vi "Main.vi"(11 "Module Admin":refnum<class "Delacor_lib_QMH_Module Admin.lvclass">) -> ()   [LabVIEW 2019, in "ManejoArchivos.lvlib"]
doc: "This template is based off of the Queued Message Handler design pattern and the Queued Message Handler project template that ships with LabVIEW.\n\nThe main difference is that the queue is private to this module and communication between modules is performed via Broadcast and Request events.\n\nRequest events are wrapped in public API methods and are handled in the Event Handling Loop (EHL) of this VI. Any module can register for Broadcast events sent by this module. The EHL generates messages based on user interface actions.\n\nThe Message Handling Loop (MHL) processes messages generated by the EHL, or by other messages. The messages are string values, so new messages can be added easily to the Message Cases case structure in the MHL. Each message cluster can also provide an optional value for Message Data, which is a variant that can be converted to whatever message-specific data is required.\n_____\nBased on DQMH Dev Tools: Project Template 7.1.0.1490."
uses:
  ManejoArchivos.lvlib
  <vilib>/Delacor/Delacor QMH/Libraries/Module Admin_class/Delacor_lib_QMH_Module Admin.lvclass
  Module Data--cluster.ctl
  Class Definitions/File/File.lvclass
  <vilib>/Delacor/Delacor QMH/Libraries/Message Queue_class/Delacor_lib_QMH_Message Queue.lvclass/Delacor_lib_QMH_Message Queue.ctl
  Stop Argument--cluster.ctl
  <vilib>/Delacor/Delacor QMH/Libraries/Module Admin_class/Delacor_lib_QMH_Module Admin.lvclass/Delacor_lib_QMH_Module Admin.ctl
  Set Column Headers Argument--cluster.ctl
  View File Argument--cluster.ctl
  Set File Path Argument--cluster.ctl
  Set File Settings Argument--cluster.ctl
  Log Data Argument--cluster.ctl
  Log Data (Reply Payload)--cluster.ctl
  Set File Format Argument--cluster.ctl
  File Formats--enum.ctl
  Close File Argument--cluster.ctl
  Get Number of Columns Argument--cluster.ctl
  Get Number of Columns (Reply Payload)--cluster.ctl
  <vilib>/Utility/miscctls.llb/LVPointTypeDef.ctl
  Class Definitions/File/File.lvclass/File.ctl
  <vilib>/Delacor/Delacor QMH/Libraries/Message Queue_class/Delacor_lib_QMH_Enqueue Message (Single).vi
  <vilib>/Delacor/Delacor QMH/Libraries/Module Admin_class/Delacor_lib_QMH_Get External Launch.vi
  Class Definitions/File/Write Column Headers.vi
  Class Definitions/File/Write File Path.vi
  Class Definitions/File/Write Save Timestamp.vi
  Class Definitions/File/Write Delimiter.vi
  Class Definitions/File/Read Column Headers.vi
  <vilib>/Delacor/Delacor QMH/Libraries/Message Queue_class/Delacor_lib_QMH_Message Queue.lvclass
panel:
  out "error out":errorcluster
  out "Status":string
  in  "Simulate MHL Error":bool
  in  "Simulate EHL Error":bool
  # "Other processes communicate with this Module via its Public API (wrappers for its Request Events).\n\nThis Module communicates with other processes via its Broadcast Events.\nAny process that wants to receive these messages can register for this module's Broadcast events."
  # "This template is for the DQMH framework. See the block diagram for more information on how to use this template."
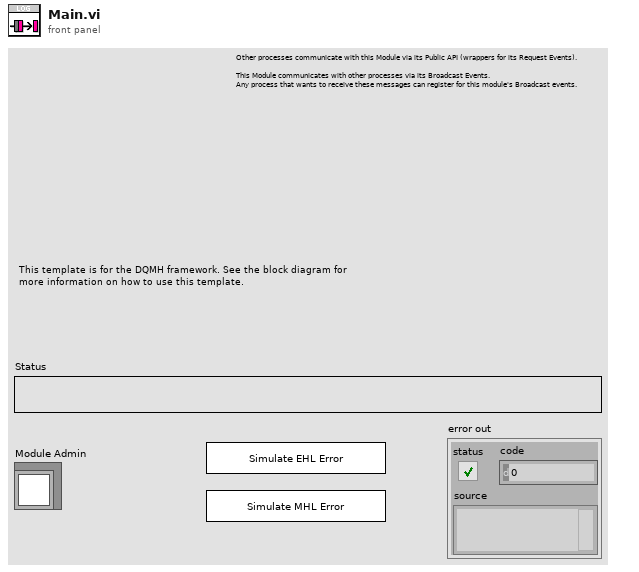
[diagram p1: front panel]
types:
  T1 = typedef "ManejoArchivos.lvlib/Request Events--cluster.ctl" = cluster{"Stop Module":refnum<user-event>, "Show Panel":refnum<user-event>, "Hide Panel":refnum<user-event>, "Get Module Execution Status":refnum<user-event>, "Show Diagram":refnum<user-event>, "Set Column Headers":refnum<user-event>, "View File":refnum<user-event>, "Set File Path":refnum<user-event>, "Set File Settings":refnum<user-event>, "Log Data":refnum<user-event>, "Set File Format":refnum<user-event>, "Close File":refnum<user-event>, "Get Number of Columns":refnum<user-event>}
  T2 = typedef "ManejoArchivos.lvlib/Module Data--cluster.ctl" = cluster{"Status":string, "File Obj":refnum<class "File.lvclass">, "View File":bool}
  T3 = enum32{"invalid lock state", "Not Locked", "Locked (No Password)", "Password-protected"}
  T4 = typedef "ManejoArchivos.lvlib/Stop Argument--cluster.ctl" = cluster{"Origin":string, "Exit via Stop Module Req?":bool, "Wait for Module to stop?":bool}
  T5 = typedef "ManejoArchivos.lvlib/Set Column Headers Argument--cluster.ctl" = cluster{"Headers":string[]}
  T6 = typedef "ManejoArchivos.lvlib/View File Argument--cluster.ctl" = cluster{"Boolean":bool}
  T7 = typedef "ManejoArchivos.lvlib/Set File Path Argument--cluster.ctl" = cluster{"Path":path}
  T8 = typedef "ManejoArchivos.lvlib/Set File Settings Argument--cluster.ctl" = cluster{"Save Time Stamp":bool, "Delimiter":enum16{"Tab", "Coma"}}
  T9 = typedef "ManejoArchivos.lvlib/Log Data Argument--cluster.ctl" = cluster{"Data":dbl[], "Wait Notifier":refnum<notifier>, "wait for reply":bool}
  T10 = typedef "ManejoArchivos.lvlib/Set File Format Argument--cluster.ctl" = cluster{"Format":T11}
  T11 = typedef "ManejoArchivos.lvlib/File Formats--enum.ctl" = enum16{"TDMS", "CSV"}
  T12 = typedef "ManejoArchivos.lvlib/Close File Argument--cluster.ctl" = cluster{"Boolean":bool}
  T13 = typedef "ManejoArchivos.lvlib/Get Number of Columns Argument--cluster.ctl" = cluster{"Wait Notifier":refnum<notifier>, "wait for reply":bool}
  T14 = typedef "LVPointTypeDef.ctl" = cluster{"Horizontal":i16, "Vertical":i16}
  T15 = enum32{"Invalid", "Standard", "Closed", "Hidden", "Minimized", "Maximized"}
  T16 = typedef "ManejoArchivos.lvlib/Log Data (Reply Payload)--cluster.ctl" = cluster{"error":errorcluster}
  T17 = typedef "ManejoArchivos.lvlib/Get Number of Columns (Reply Payload)--cluster.ctl" = cluster{"error":errorcluster, "Number Of Columns":i32}
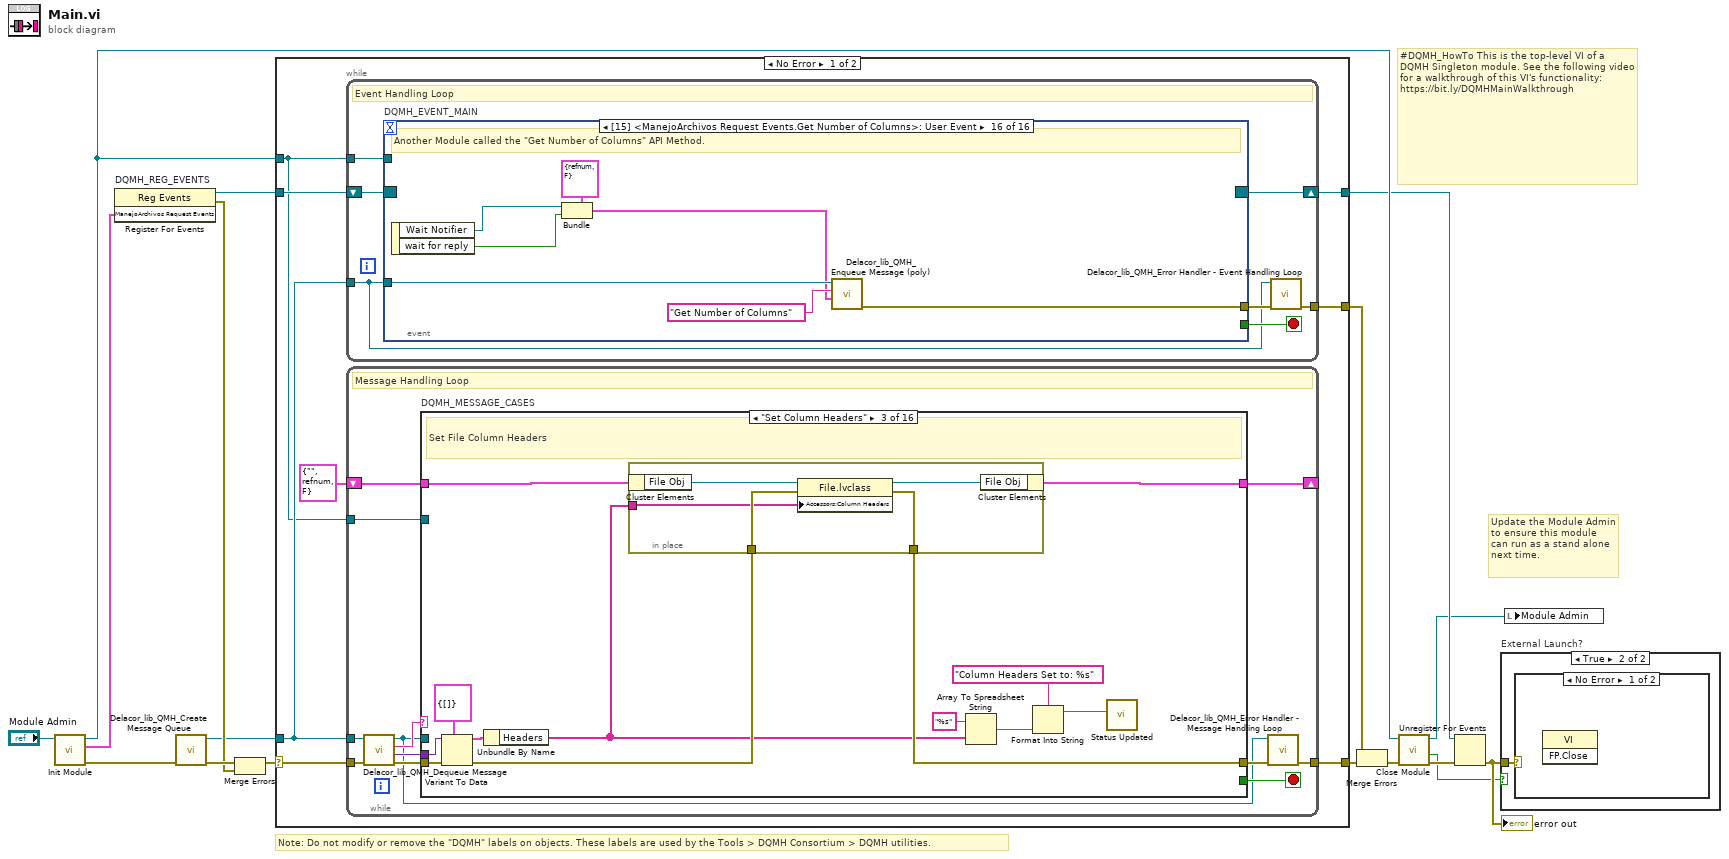
[diagram p0: block diagram]
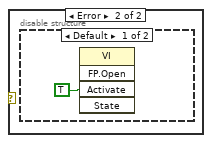
[diagram p3: hidden frame]
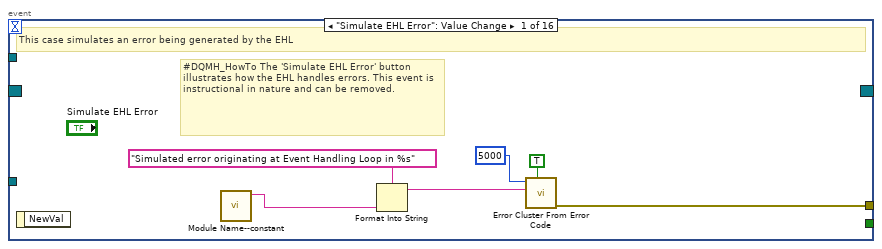
[diagram p5: hidden frame]
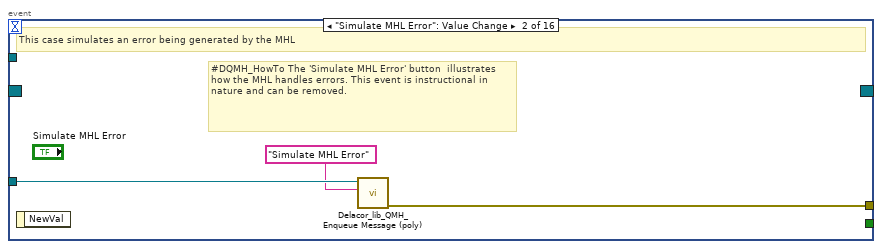
[diagram p6: hidden frame]
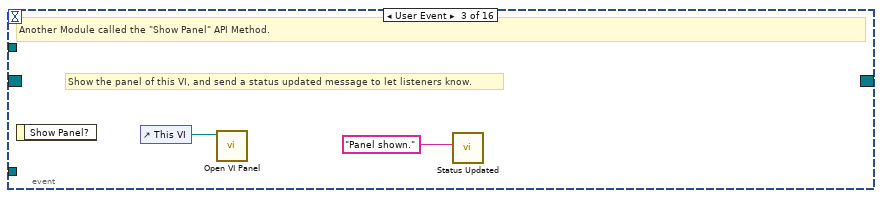
[diagram p7: hidden frame]
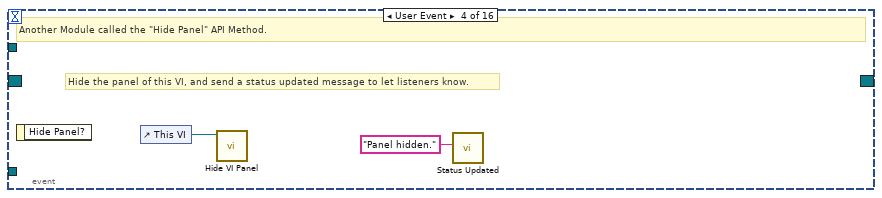
[diagram p8: hidden frame]
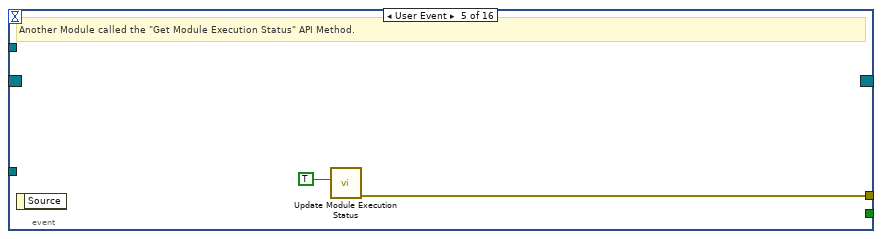
[diagram p9: hidden frame]
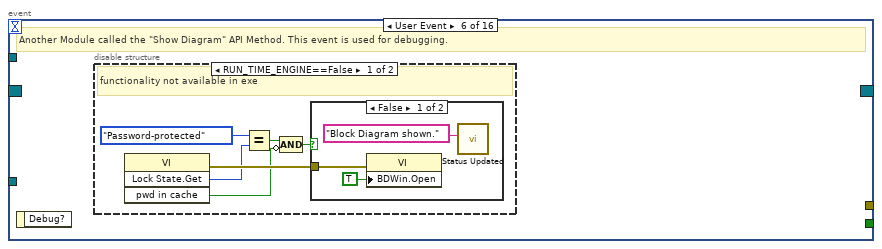
[diagram p10: hidden frame]
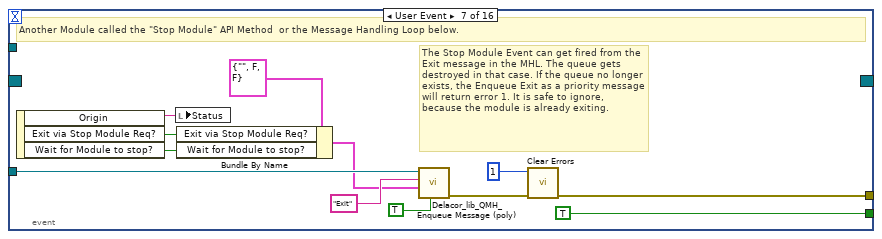
[diagram p13: hidden frame]
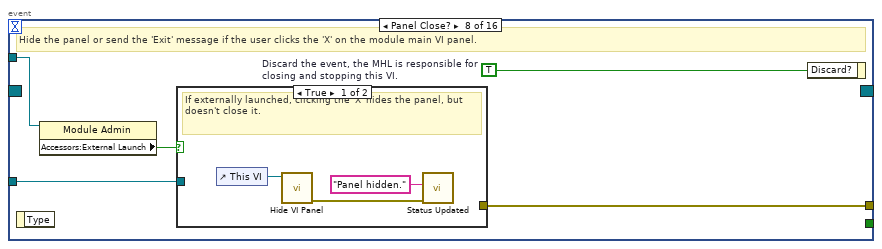
[diagram p14: hidden frame]
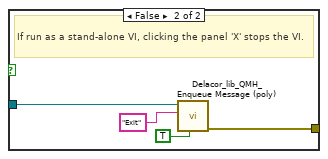
[diagram p15: hidden frame]
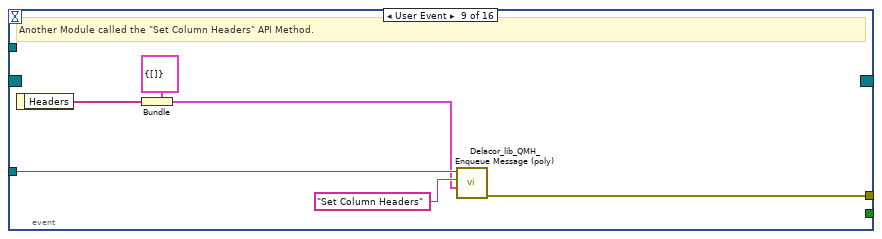
[diagram p16: hidden frame]
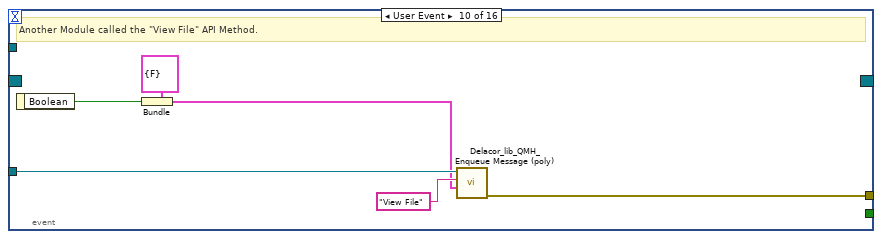
[diagram p17: hidden frame]
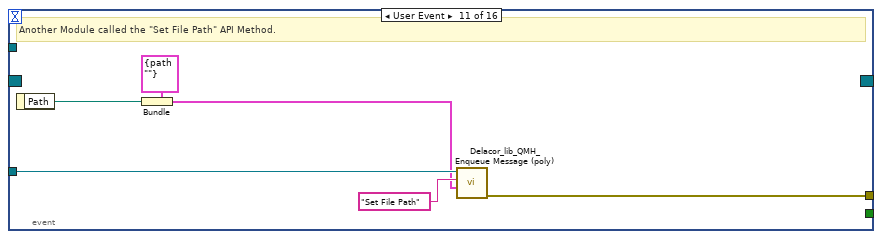
[diagram p18: hidden frame]
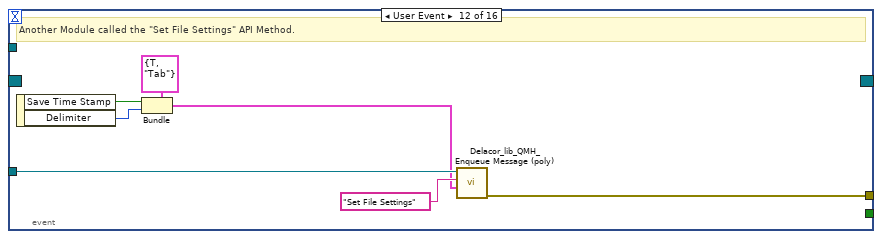
[diagram p19: hidden frame]
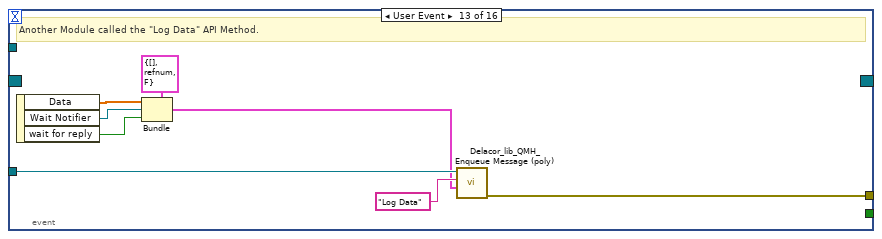
[diagram p20: hidden frame]
diagram:
  # "#DQMH_HowTo This is the top-level VI of a DQMH Singleton module. See the following video for a walkthrough of this VI's functionality: https://bit.ly/DQMHMainWalkthrough"
  # "Note: Do not modify or remove the \"DQMH\" labels on objects. These labels are used by the Tools > DQMH Consortium > DQMH utilities."
  # "Update the Module Admin to ensure this module can run as a stand alone next time."
  n1 = call "Init Module.vi"("Singleton Module Admin in"="Module Admin") -> ("error out"=w16:errorcluster, "ManejoArchivos Request Events"=w5:T1, "Singleton Module Admin out"=w8:refnum<class "Delacor_lib_QMH_Module Admin.lvclass">)  [unwired: 8 in]
  n2 = register-events "DQMH_REG_EVENTS"(w5) -> (reference out=w6:refnum<event-registration>, error out=w9:errorcluster)  [unwired: 2 in]
  n3 = call <vilib>:"Delacor_lib_QMH_Create Message Queue.vi"("error in"=w16) -> ("error out"=w11:errorcluster, "Message Queue"=w4:refnum<class "Delacor_lib_QMH_Message Queue.lvclass">)  [unwired: 9 in]
  n4 = Merge Errors(w11, w9) -> (w10:errorcluster)
  n5 = case shown="No Error" w10 {
    selector: w10 -> [w23 w357]
    tunnel: [w25 w356] -> w17
    tunnel: [w22 w355] -> w7
    tunnel: w6 -> [w20 w355]
    tunnel: w4 -> [w19 w350]
    tunnel: [w24 _] -> w14
    tunnel: w8 -> [w18 w351]
    frame No Error {
      n6 = while {
        tunnel: w19 -> [w26]
        shift-right: [w29] -> w22
        shift-left: w20 -> [w30]
        tunnel: [w31] -> w24
        tunnel: w18 -> [w27]
        stop <- w28 stop-if-true
        # "Event Handling Loop"
        n7 = event "DQMH_EVENT_MAIN" shown="[15] <ManejoArchivos Request Events.Get Number of Columns>: User Event" {
          selector: w30 -> [_ _ _ _ _ _ _ _ _ _ _ _ _ _ _ _]
          dyn-events: [_ _ _ _ _ _ _ _ _ _ _ _ _ _ _ _] -> w29
          timeout: _ -> [_ _ _ _ _ _ _ _ _ _ _ _ _ _ _ _]
          tunnel: [_ _ _ _ _ _ TRUE ("Discard?") _ _ _ _ _ _ _ _ _] -> w28
          tunnel: w26 -> [_ w40 _ _ _ _ w64 w71 w86 w92 w98 w105 w113 w119 w125 w132]
          tunnel: [w38 w41 _ _ w47 _ w67 w73 w81 w87 w93 w99 w108 w114 w120 w128] -> w32
          tunnel: w27 -> [_ _ _ _ _ _ _ w70 _ _ _ _ _ _ _ _]
          event "Simulate EHL Error": Value Change {
            # "#DQMH_HowTo The 'Simulate EHL Error' button  illustrates how the EHL handles errors. This event is instructional in nature and can be removed."
            # "This case simulates an error being generated by the EHL"
            n8 = event-data() -> ()  [unwired: 1 in, 1 out]
            n9 = call "Module Name--constant.vi"() -> ("Module Name"=w35:string)  [unwired: 11 in]
            n10 = Format Into String(format string="Simulated error originating at Event Handling Loop in %s", w35) -> (resulting string=w36:string)  [unwired: 2 in, 1 out]
            n11 = call <vilib>:"Error Cluster From Error Code.vi"("show call chain? (False)"=TRUE, "error message (\"\")"=w36, "error code (0)"=5000) -> ("error out"=w38:errorcluster)  [unwired: 6 in]
          }
          event "Simulate MHL Error": Value Change {
            # "#DQMH_HowTo The 'Simulate MHL Error' button  illustrates how the MHL handles errors. This event is instructional in nature and can be removed."
            # "This case simulates an error being generated by the MHL"
            n12 = event-data() -> ()  [unwired: 1 in, 1 out]
            n13 = call-poly <vilib>:"Delacor_lib_QMH_Enqueue Message (poly).vi"("Message"="Simulate MHL Error", "Message Queue in"=w40) -> ("error out"=w41:errorcluster)  [unwired: 8 in, 1 out]
          }
          event User Event {
            # "Show the panel of this VI, and send a status updated message to let listeners know."
            # "Another Module called the \"Show Panel\" API Method."
            n14 = event-data() -> ()  [unwired: 1 in, 1 out]
            n15 = control-ref of="This VI"() -> (w43:refnum<vi>)
            n16 = call "Open VI Panel.vi"("VI"=w43) -> ()  [unwired: 10 in, 1 out]
            n17 = call "Status Updated.vi"("Status"="Panel shown." ("format string")) -> ()  [unwired: 10 in, 1 out]
          }
          event User Event {
            # "Hide the panel of this VI, and send a status updated message to let listeners know."
            # "Another Module called the \"Hide Panel\" API Method."
            n18 = event-data() -> ()  [unwired: 1 in, 1 out]
            n19 = control-ref of="This VI"() -> (w45:refnum<vi>)
            n20 = call "Hide VI Panel.vi"("VI"=w45) -> ()  [unwired: 10 in, 1 out]
            n21 = call "Status Updated.vi"("Status"="Panel hidden." ("format string")) -> ()  [unwired: 10 in, 1 out]
          }
          event User Event {
            # "Another Module called the \"Get Module Execution Status\" API Method."
            n22 = event-data() -> ()  [unwired: 1 in, 1 out]
            n23 = call "Update Module Execution Status.vi"("Running?"=TRUE) -> ("error out"=w47:errorcluster)  [unwired: 10 in]
          }
          event User Event {
            # "Another Module called the \"Show Diagram\" API Method. This event is used for debugging."
            n24 = event-data() -> ()  [unwired: 1 in, 1 out]
            n25 = disable-structure shown="RUN_TIME_ENGINE==False" {
              frame condition #0 (active) {
                # "functionality not available in exe"
                n26 = invoke on="Invoke Node" class="VI" method="Lock State.Get"() -> (error out=w53:errorcluster, "Get Lock State"=w52:T3, "pwd in cache"=w49:bool)  [unwired: 4 in, 1 out]
                n27 = Equal?(x=T3."Password-protected", y=w52) -> (x = y?=w50:bool)
                n28 = Compound Arithmetic op=AND(w50, invert w49) -> (w48:bool)
                n29 = case shown="False" w48 {
                  tunnel: w53 -> [w56 _]
                  frame False {
                    n30 = property on="Property Node" class="VI"(error in=w56, "BDWin.Open"=TRUE ("Block Diagram Window:Open")) -> ()  [unwired: 1 in, 2 out]
                    n31 = call "Status Updated.vi"("Status"="Block Diagram shown." ("format string")) -> ()  [unwired: 10 in, 1 out]
                  }
                  frame True {
                    # "Password-protected VI, and the password is not in the cache. Do not show the diagram."
                  }
                }
              }
              frame condition #1 {
              }
            }
          }
          event User Event {
            # "The Stop Module Event can get fired from the Exit message in the MHL. The queue gets destroyed in that case. If the queue no longer exists, the Enqueue Exit as a priority message will return error 1. It is safe to ignore, because the module is already exiting."
            # "Another Module called the \"Stop Module\" API Method  or the Message Handling Loop below."
            n32 = event-data() -> ("Origin"=w63:string, "Exit via Stop Module Req?"=w59:bool, "Wait for Module to stop?"=w58:bool)  [unwired: 1 in]
            n33 = local write "Status"(w63) -> ()
            n34 = Bundle By Name(cluster=T4 {"Origin"="", "Exit via Stop Module Req?"=FALSE, "Wait for Module to stop?"=FALSE} ("Stop Argument"), "Exit via Stop Module Req?"=w59, "Wait for Module to stop?"=w58) -> (w57:T4)
            n35 = call-poly <vilib>:"Delacor_lib_QMH_Enqueue Message (poly).vi"("Priority Message? (F)"=TRUE, "Message Data"=w57, "Message"="Exit", "Message Queue in"=w64) -> ("error out"=w68:errorcluster)  [unwired: 6 in, 1 out]
            n36 = call <vilib>:"Clear Errors.vi"("error in (no error)"=w68, "specific error code to clear (0: all)"=1) -> ("error out"=w67:errorcluster)  [unwired: 4 in, 1 out]
          }
          event Panel Close? {
            w72 = TRUE  # Discard the event, the MHL is responsible for closing and stopping this VI.
            # "Hide the panel or send the 'Exit' message if the user clicks the 'X' on the module main VI panel."
            n37 = event-data() -> ()  [unwired: 1 in, 1 out]
            n38 = property on="Property Node" class="Module Admin"(reference=w70) -> ("Accessors:External Launch"=w69:bool)  [unwired: 1 in, 2 out]
            n39 = case shown="True" w69 {
              tunnel: w71 -> [_ w79]
              tunnel: [_ w80] -> w73
              frame True {
                # "If externally launched, clicking the 'X' hides the panel, but doesn't close it."
                n40 = control-ref of="This VI"() -> (w76:refnum<vi>)
                n41 = call "Hide VI Panel.vi"("VI"=w76) -> ("error out"=w74:errorcluster)  [unwired: 10 in]
                n42 = call "Status Updated.vi"("error in"=w74, "Status"="Panel hidden." ("format string")) -> ()  [unwired: 9 in, 1 out]
              }
              frame False {
                # "If run as a stand-alone VI, clicking the panel 'X' stops the VI."
                n43 = call-poly <vilib>:"Delacor_lib_QMH_Enqueue Message (poly).vi"("Priority Message? (F)"=TRUE, "Message"="Exit", "Message Queue in"=w79) -> ("error out"=w80:errorcluster)  [unwired: 7 in, 1 out]
              }
            }
            n44 = event-data ("Event Filter Node")("Discard?"=w72) -> ()  [unwired: 1 in, 1 out]
          }
          event User Event {
            # "Another Module called the \"Set Column Headers\" API Method."
            n45 = event-data() -> ("Headers"=w82:string[])  [unwired: 1 in]
            n46 = Bundle(cluster=T5 {"Headers"=[]} ("Set Column Headers Argument"), "Headers"=w82) -> (w83:T5)
            n47 = call-poly <vilib>:"Delacor_lib_QMH_Enqueue Message (poly).vi"("Message Data"=w83, "Message"="Set Column Headers", "Message Queue in"=w86) -> ("error out"=w81:errorcluster)  [unwired: 7 in, 1 out]
          }
          event User Event {
            # "Another Module called the \"View File\" API Method."
            n48 = event-data() -> ("Boolean"=w88:bool)  [unwired: 1 in]
            n49 = Bundle(cluster=T6 {"Boolean"=FALSE} ("View File Argument"), "Boolean"=w88) -> (w89:T6)
            n50 = call-poly <vilib>:"Delacor_lib_QMH_Enqueue Message (poly).vi"("Message Data"=w89, "Message"="View File", "Message Queue in"=w92) -> ("error out"=w87:errorcluster)  [unwired: 7 in, 1 out]
          }
          event User Event {
            # "Another Module called the \"Set File Path\" API Method."
            n51 = event-data() -> ("Path"=w94:path)  [unwired: 1 in]
            n52 = Bundle(cluster=T7 {"Path"=path ""} ("Set File Path Argument"), "Path"=w94) -> (w95:T7)
            n53 = call-poly <vilib>:"Delacor_lib_QMH_Enqueue Message (poly).vi"("Message Data"=w95, "Message"="Set File Path", "Message Queue in"=w98) -> ("error out"=w93:errorcluster)  [unwired: 7 in, 1 out]
          }
          event User Event {
            # "Another Module called the \"Set File Settings\" API Method."
            n54 = event-data() -> ("Save Time Stamp"=w101:bool, "Delimiter"=w100:enum16{"Tab", "Coma"})  [unwired: 1 in]
            n55 = Bundle(cluster=T8 {"Save Time Stamp"=TRUE, "Delimiter"=enum."Tab"} ("Set File Settings Argument"), "Save Time Stamp"=w101, "Delimiter"=w100) -> (w102:T8)
            n56 = call-poly <vilib>:"Delacor_lib_QMH_Enqueue Message (poly).vi"("Message Data"=w102, "Message"="Set File Settings", "Message Queue in"=w105) -> ("error out"=w99:errorcluster)  [unwired: 7 in, 1 out]
          }
          event User Event {
            # "Another Module called the \"Log Data\" API Method."
            n57 = event-data() -> ("Data"=w109:dbl[], "Wait Notifier"=w107:refnum<notifier>, "wait for reply"=w106:bool)  [unwired: 1 in]
            n58 = Bundle(cluster=T9 {"Data"=[], "Wait Notifier"=refnum, "wait for reply"=FALSE} ("Log Data Argument"), "Data"=w109, "Wait Notifier"=w107, "wait for reply"=w106) -> (w110:T9)
            n59 = call-poly <vilib>:"Delacor_lib_QMH_Enqueue Message (poly).vi"("Message Data"=w110, "Message"="Log Data", "Message Queue in"=w113) -> ("error out"=w108:errorcluster)  [unwired: 7 in, 1 out]
          }
          event User Event {
            # "Another Module called the \"Set File Format\" API Method."
            n60 = event-data() -> ("Format"=w115:T11)  [unwired: 1 in]
            n61 = Bundle(cluster=T10 {"Format"=enum."TDMS"} ("Set File Format Argument"), "Format"=w115) -> (w116:T10)
            n62 = call-poly <vilib>:"Delacor_lib_QMH_Enqueue Message (poly).vi"("Message Data"=w116, "Message"="Set File Format", "Message Queue in"=w119) -> ("error out"=w114:errorcluster)  [unwired: 7 in, 1 out]
          }
          event User Event {
            # "Another Module called the \"Close File\" API Method."
            n63 = event-data() -> ("Boolean"=w121:bool)  [unwired: 1 in]
            n64 = Bundle(cluster=T12 {"Boolean"=FALSE} ("Close File Argument"), "Boolean"=w121) -> (w122:T12)
            n65 = call-poly <vilib>:"Delacor_lib_QMH_Enqueue Message (poly).vi"("Message Data"=w122, "Message"="Close File", "Message Queue in"=w125) -> ("error out"=w120:errorcluster)  [unwired: 7 in, 1 out]
          }
          event User Event {
            # "Another Module called the \"Get Number of Columns\" API Method."
            n66 = event-data() -> ("Wait Notifier"=w127:refnum<notifier>, "wait for reply"=w126:bool)  [unwired: 1 in]
            n67 = Bundle(cluster=T13 {"Wait Notifier"=refnum, "wait for reply"=FALSE} ("Get Number of Columns Argument"), "Wait Notifier"=w127, "wait for reply"=w126) -> (w129:T13)
            n68 = call-poly <vilib>:"Delacor_lib_QMH_Enqueue Message (poly).vi"("Message Data"=w129, "Message"="Get Number of Columns", "Message Queue in"=w132) -> ("error out"=w128:errorcluster)  [unwired: 7 in, 1 out]
          }
        }
        n69 = call-dynamic "Delacor_lib_QMH_Error Handler - Event Handling Loop.vi"("error in"=w32, "Message Queue in"=w26) -> ("dup error in"=w31:errorcluster)  [unwired: 8 in, 1 out]
      }
      n70 = while {
        tunnel: w19 -> [w133]
        shift-right: [w141] -> _
        shift-left: T2 {"Status"="", "File Obj"=refnum, "View File"=FALSE} ("Data Cluster") -> [w142]
        tunnel: w23 -> [w144]
        tunnel: [w136] -> w25
        tunnel: w18 -> [w137]
        stop <- w140 stop-if-true
        # "Message Handling Loop"
        n71 = call-dynamic "Delacor_lib_QMH_Dequeue Message.vi"("error in"=w144, "Message Queue in"=w133) -> ("error out"=w143:errorcluster, "Message Data"=w138:variant, "Message"=w139:string, "Message Queue out"=w134:refnum<class "Delacor_lib_QMH_Message Queue.lvclass">)  [unwired: 6 in]
        n72 = case "DQMH_MESSAGE_CASES" shown="\"Set Column Headers\"" w139 {
          selector: w139 -> [_ _ _ _ _ _ _ _ _ _ _ _ _ _ _ w345]
          tunnel: w134 -> [_ _ _ _ _ _ _ _ _ _ _ _ _ w305 w330 _]
          tunnel: w143 -> [w162 w166 w179 w193 w204 w220 w236 w245 w263 w285 w290 w292 w301 w312 w336 w348]
          tunnel: [w160 w166 w172 w188 w197 w219 w235 w239 w255 w276 w289 w292 w300 w308 w331 w349] -> w135
          tunnel: w142 -> [w151 w165 w175 w189 w200 w215 w230 w240 w254 w275 w288 w291 w298 w307 w322 w346]
          tunnel: [w150 w165 w174 w187 w199 w214 w231 w240 w253 w275 w288 w291 w298 w307 w322 w346] -> w141
          tunnel: [_ _ _ _ _ _ _ _ _ _ _ _ _ _ w329 _] -> w140
          tunnel: w138 -> [_ _ w178 w192 w203 w218 w234 w243 w262 w283 _ _ _ w306 w328 _]
          tunnel: w137 -> [w152 _ _ _ _ _ _ _ _ _ _ _ _ w304 w323 _]
          frame "Initialize" {
            w146 = "Initial Message" ("Initial Message")
            # "#DQMH_CodeNeeded - Initialize the appearance of the front panel."
            # "#DQMH_CodeNeeded - Initialize your state data here."
            # "Initialize - Any operation that needs to be done before the module can receive messages. Synchronize Caller Events.vi will inform Start Module.vi that the module has launched and is ready to receive messages. Module Did Init.vi will broadcast that the module initialized."
            n73 = call "Synchronize Caller Events.vi"("error in"=w162, "Singleton Module Admin in"=w152) -> ("error out"=w161:errorcluster, "Singleton Module Admin out"=w147:refnum<class "Delacor_lib_QMH_Module Admin.lvclass">)  [unwired: 8 in]
            n74 = property on="Property Node" class="Module Admin"(reference=w147) -> ("Accessors:External Launch"=w156:bool)  [unwired: 1 in, 2 out]
            n75 = Select(t=T15."Hidden" ("State"), s=w156, f=T15."Standard" ("State")) -> (s? t:f=w153:T15)
            n76 = call "Module Name--constant.vi"() -> ("Module Name"=w159:string)  [unwired: 11 in]
            n77 = property on="Property Node" class="VI"("Front Panel.Title"=w159) -> (reference out=w158:refnum<vi>, error out=w164:errorcluster)  [unwired: 2 in]
            n78 = invoke on="Invoke Node" class="VI" method="FP.Open"(reference=w158, error in=w164, "State"=w153) -> (reference out=w157:refnum<vi>, error out=w163:errorcluster)  [unwired: 2 in, 3 out]
            n79 = Bundle By Name(cluster=w151, "Status"=w146) -> (w150:T2)
            n80 = invoke on="Invoke Node" class="VI" method="FP.Center"(reference=w157, error in=w163) -> ()  [unwired: 1 in, 3 out]
            n81 = property on="Pane" class="Pane"("Origin"=T14 {"Horizontal"=0, "Vertical"=0}) -> ()  [unwired: 2 in, 2 out]
            n82 = call "Module Name--constant.vi"() -> ("Module Name"=w148:string)  [unwired: 11 in]
            n83 = call "Module Did Init.vi"("error in"=w161, "Initialized?"=TRUE, "Origin"=w148) -> ("error out"=w160:errorcluster)  [unwired: 8 in]
            "Status" <- w146
          }
          frame "---Module Specific---" {
            # "Separator -- The following cases handle messages specific to this Module."
          }
          frame "Set Column Headers" {
            # "Set File Column Headers"
            n84 = Variant To Data(error in=w179, type=T5 {"Headers"=[]} ("Set Column Headers Argument"), Variant=w178) -> (data=w176:T5, error out=w173:errorcluster)
            n85 = Unbundle By Name(w176) -> ("Headers"=w171:string[])
            n86 = in-place {
              in-place-border: w173 -> [w184]
              in-place-border: [w183] -> w172
              in-place-border: w171 -> [w180]
              n87 = in-place-cluster #1(w175) -> ("File Obj"=w182:refnum<class "File.lvclass">)
              n88 = property class="File.lvclass"(reference=w182, error in=w184, "Accessors:Column Headers"=w180) -> (reference out=w181:refnum<class "File.lvclass">, error out=w183:errorcluster)
              n89 = in-place-cluster #1("File Obj"=w181) -> (w174:T2)
            }
            n90 = Array To Spreadsheet String(array=w171, 3:"%s" ("format string")) -> (spreadsheet string=w168:string)  [unwired: 1 in]
            n91 = Format Into String(format string="Column Headers Set to: %s" ("Status"), w168) -> (resulting string=w169:string)  [unwired: 2 in, 1 out]
            n92 = call "Status Updated.vi"("Status"=w169) -> ()  [unwired: 10 in, 1 out]
          }
          frame "View File" {
            # "View File"
            n93 = Variant To Data(error in=w193, type=T6 {"Boolean"=FALSE} ("View File Argument"), Variant=w192) -> (data=w190:T6, error out=w188:errorcluster)
            n94 = Unbundle By Name(w190) -> ()  [unwired: 1 out]
            n95 = Bundle By Name(cluster=w189, "View File"=TRUE) -> (w187:T2)
            n96 = call "Status Updated.vi"("Status"="View File at the end set to true") -> ()  [unwired: 10 in, 1 out]
          }
          frame "Set File Path" {
            # "Set File Path"
            n97 = Variant To Data(error in=w204, type=T7 {"Path"=path ""} ("Set File Path Argument"), Variant=w203) -> (data=w201:T7, error out=w198:errorcluster)
            n98 = Unbundle By Name(w201) -> ("Path"=w196:path)
            n99 = in-place {
              in-place-border: w198 -> [w209]
              in-place-border: w196 -> [w205]
              in-place-border: [w208] -> w197
              n100 = in-place-cluster #2(w200) -> ("File Obj"=w207:refnum<class "File.lvclass">)
              n101 = property class="File.lvclass"(reference=w207, error in=w209, "Accessors:File Path"=w205) -> (reference out=w206:refnum<class "File.lvclass">, error out=w208:errorcluster)
              n102 = in-place-cluster #2("File Obj"=w206) -> (w199:T2)
            }
            n103 = Format Into String(format string="File path Set to: %s", w196) -> (resulting string=w195:string)  [unwired: 2 in, 1 out]
            n104 = call "Status Updated.vi"("Status"=w195) -> ()  [unwired: 10 in, 1 out]
          }
          frame "Set File Settings" {
            # "Set File Settings"
            n105 = Variant To Data(error in=w220, type=T8 {"Save Time Stamp"=TRUE, "Delimiter"=enum."Tab"} ("Set File Settings Argument"), Variant=w218) -> (data=w216:T8, error out=w219:errorcluster)
            n106 = Unbundle By Name(w216) -> ("Save Time Stamp"=w213:bool, "Delimiter"=w212:enum16{"Tab", "Coma"})
            n107 = in-place {
              in-place-border: w213 -> [w222]
              in-place-border: w212 -> [w221]
              n108 = in-place-cluster #3(w215) -> ("File Obj"=w224:refnum<class "File.lvclass">)
              n109 = property class="File.lvclass"(reference=w224, "Accessors:Save Timestamp"=w222, "Accessors:Delimiter"=w221) -> (reference out=w223:refnum<class "File.lvclass">)  [unwired: 1 in, 1 out]
              n110 = in-place-cluster #3("File Obj"=w223) -> (w214:T2)
            }
            n111 = Format Into String(format string="File Settings set to: Save timestamp =%s, Delimiter = %s", w213, w212) -> (resulting string=w211:string)  [unwired: 2 in, 1 out]
            n112 = call "Status Updated.vi"("Status"=w211) -> ()  [unwired: 10 in, 1 out]
          }
          frame "Set File Format" {
            # "Set File Format"
            n113 = Variant To Data(error in=w236, type=T10 {"Format"=enum."TDMS"} ("Set File Format Argument"), Variant=w234) -> (data=w232:T10, error out=w235:errorcluster)
            n114 = Unbundle By Name(w232) -> ("Format"=w227:T11)
            n115 = Format Into String(format string="Format File set to: %s", w227) -> (resulting string=w229:string)  [unwired: 2 in, 1 out]
            n116 = call "Status Updated.vi"("Status"=w229) -> ()  [unwired: 10 in, 1 out]
            n117 = Unbundle By Name(w230) -> ("File Obj"=w226:refnum<class "File.lvclass">)
            n118 = call "Preserving Class Values.vi"("Format"=w227, "File in"=w226) -> ("File out"=w225:refnum<class "File.lvclass">)  [unwired: 9 in]
            n119 = Bundle By Name(cluster=w230, "File Obj"=w225) -> (w231:T2)
          }
          frame "Close File" {
            n120 = Variant To Data(error in=w245, type=T12 {"Boolean"=FALSE} ("Close File Argument"), Variant=w243) -> (data=w241:T12, error out=w244:errorcluster)
            n121 = Unbundle By Name(w241) -> ()  [unwired: 1 out]
            n122 = Unbundle By Name(w240) -> ("File Obj"=w238:refnum<class "File.lvclass">)
            n123 = call-dynamic "Close File.vi"("error in (no error)"=w244, "File in"=w238) -> ("error out"=w239:errorcluster)  [unwired: 8 in, 1 out]
            n124 = call "Status Updated.vi"("Status"="File Closed") -> ()  [unwired: 10 in, 1 out]
          }
          frame "Log Data" {
            # "Log data to file"
            n125 = Variant To Data(error in=w263, type=T9 {"Data"=[], "Wait Notifier"=refnum, "wait for reply"=FALSE} ("Log Data Argument"), Variant=w262) -> (data=w260:T9, error out=w250:errorcluster)
            n126 = Unbundle By Name(w260) -> ("Data"=w251:dbl[], "Wait Notifier"=w259:refnum<notifier>, "wait for reply"=w258:bool)
            n127 = in-place {
              in-place-border: w250 -> [w266]
              in-place-border: w251 -> [w265]
              in-place-border: [w264] -> w252
              n128 = in-place-cluster #4(w254) -> ("File Obj"=w268:refnum<class "File.lvclass">)
              n129 = call-dynamic "Log Data.vi"("error in (no error)"=w266, "Data"=w265, "File in"=w268) -> ("error out"=w264:errorcluster, "File out"=w267:refnum<class "File.lvclass">)  [unwired: 7 in]
              n130 = in-place-cluster #4("File Obj"=w267) -> (w253:T2)
            }
            n131 = feedback #5() -> (w247:dbl)  [unwired: 1 in]
            n132 = Increment(x=w247) -> (x+1=w246:dbl)
            n133 = feedback-in #5(w246) -> ()
            n134 = Format Into String(format string="Data logged into file (%d)", w246) -> (resulting string=w249:string)  [unwired: 2 in, 1 out]
            n135 = call "Status Updated.vi"("Status"=w249) -> ()  [unwired: 10 in, 1 out]
            n136 = Bundle By Name(cluster=T16 {"error"={"status"=FALSE, "code"=0, "source"=""}} ("Log Data (Reply Payload)"), "error"=w252) -> (w257:T16)
            n137 = Merge Errors(w250, w252) -> (w255:errorcluster)
            n138 = case "DQMH_FIRE_NOTIFIER" shown="True" w258 {
              tunnel: w259 -> [_ w270]
              tunnel: w257 -> [_ w269]
              frame False {
              }
              frame True {
                n139 = Send Notification(notification=w269, notifier=w270) -> ()  [unwired: 1 in, 2 out]
              }
            }
          }
          frame "Get Number of Columns" {
            n140 = Variant To Data(error in=w285, type=T13 {"Wait Notifier"=refnum, "wait for reply"=FALSE} ("Get Number of Columns Argument"), Variant=w283) -> (data=w281:T13, error out=w284:errorcluster)
            n141 = Unbundle By Name(w281) -> ("Wait Notifier"=w280:refnum<notifier>, "wait for reply"=w279:bool)
            n142 = Unbundle By Name(w275) -> ("File Obj"=w274:refnum<class "File.lvclass">)
            n143 = property class="File.lvclass"(reference=w274) -> ("Accessors:Column Headers"=w273:string[])  [unwired: 1 in, 2 out]
            n144 = Array Size(array=w273) -> (size(s)=w272:i32)
            n145 = Bundle By Name(cluster=T17 {"error"={"status"=FALSE, "code"=0, "source"=""}, "Number Of Columns"=0} ("Get Number of Columns (Reply Payload)"), "Number Of Columns"=w272) -> (w278:T17)
            n146 = call "Status Updated.vi"("Status"="Number of columns retrieved from Module") -> ()  [unwired: 10 in, 1 out]
            n147 = Merge Errors(w284) -> (w276:errorcluster)
            n148 = case "DQMH_FIRE_NOTIFIER" shown="True" w279 {
              tunnel: w280 -> [_ w287]
              tunnel: w278 -> [_ w286]
              frame False {
              }
              frame True {
                n149 = Send Notification(notification=w286, notifier=w287) -> ()  [unwired: 1 in, 2 out]
              }
            }
          }
          frame "---Copy This Frame---" {
            # "Duplicate this frame when creating new messages.  Change this comment in the duplicated frame to describe this message."
            n150 = Merge Errors(w290) -> (w289:errorcluster)
          }
          frame "---Exit and Error Handling---" {
            # "Separator - The following cases handle errors and exit messages."
          }
          frame "Simulate MHL Error" {
            # "#DQMH_HowTo The 'Simulate MHL Error' button  illustrates how the MHL handles errors. This event is instructional in nature and can be removed."
            # "Simulate an error occurring at the MHL"
            n151 = call "Module Name--constant.vi"() -> ("Module Name"=w294:string)  [unwired: 11 in]
            n152 = Format Into String(format string="Simulated error originating at Message Handling Loop in %s", w294) -> (resulting string=w295:string)  [unwired: 2 in, 1 out]
            n153 = call <vilib>:"Error Cluster From Error Code.vi"("show call chain? (False)"=TRUE, "error message (\"\")"=w295, "error code (0)"=5001) -> ("error out"=w299:errorcluster)  [unwired: 6 in]
            n154 = Merge Errors(w301, w299) -> (w300:errorcluster)
          }
          frame "Error" {
            # "#DQMH_CodeRecommended - If the module is running in standalone mode (External Launch = FALSE), this code will pop up an error dialog and call the 'Exit' message if an error occurs. Add more fine-grained error management here."
            # "Error - Check the error message data and respond accordingly. This message is sent by the \"Error Handler\" VIs at the end of each loop in this application."
            n155 = property on="Property Node" class="Module Admin"(reference=w304) -> ("Accessors:External Launch"=w303:bool)  [unwired: 1 in, 2 out]
            n156 = Variant To Data(error in=w312, type=errorcluster {"status"=FALSE, "code"=0, "source"=""} ("error constant"), Variant=w306) -> (data=w302:errorcluster, error out=w310:errorcluster)
            n157 = local write "error out"(w302) -> ()
            n158 = call "Error Reported.vi"("Error"=w302) -> ()  [unwired: 10 in, 1 out]
            n159 = case shown="False" w303 {
              tunnel: [w317 _] -> w309
              tunnel: w305 -> [w315 _]
              tunnel: w302 -> [w316 _]
              frame False {
                n160 = disable-structure shown="Default" {
                  disable-tunnel: w316 -> [w318 _]
                  frame condition #0 (active) {
                    # "If the module is running standalone, then pop up an error dialog and call the \"Exit\" message."
                    n161 = call <vilib>:"Simple Error Handler.vi"("error in (no error)"=w318) -> ()  [unwired: 4 in, 5 out]
                  }
                  frame condition #1 {
                    # "To prevent the Simple Error Handler VI from being loaded (e.g. when deploying to a Real-Time target), add the Conditional Disable Symbol \"DQMH_Disable_SEH\" to your project and set it to TRUE."
                  }
                }
                n162 = call-poly <vilib>:"Delacor_lib_QMH_Enqueue Message (poly).vi"("Priority Message? (F)"=TRUE, "Message"="Exit", "Message Queue in"=w315) -> ("error out"=w317:errorcluster)  [unwired: 7 in, 1 out]
              }
              frame True {
                # "If the module was launched externally, calling the Error Reported broadcast VI is the only action performed by the \"Error\" message. The module's caller can then process the error appropriately."
              }
            }
            n163 = Merge Errors(w310, w309) -> (w308:errorcluster)
          }
          frame "Exit" {
            w327 = 91  # 91: not all Exit messages will have an argument
            w329 = TRUE  # Stop the VI
            # "Release the message queue reference"
            # "#DQMH_CodeNeeded - Add any required cleanup code here."
            # "Exit - Exit the application."
            n164 = Variant To Data(error in=w336, type=T4 {"Origin"="", "Exit via Stop Module Req?"=FALSE, "Wait for Module to stop?"=FALSE} ("Stop Argument"), Variant=w328) -> (data=w325:T4, error out=w333:errorcluster)
            n165 = call <vilib>:"Clear Errors.vi"("error in (no error)"=w333, "specific error code to clear (0: all)"=w327) -> ("error out"=w335:errorcluster)  [unwired: 4 in, 1 out]
            n166 = control-ref of="This VI"() -> (w324:refnum<vi>)
            n167 = call-dynamic "Delacor_lib_QMH_Release Message Queue.vi"("error in"=w335, "Message Queue"=w330) -> ("error out"=w334:errorcluster)  [unwired: 9 in]
            n168 = call "Handle Exit.vi"("Stop Argument"=w325, "Admin in"=w323, "VI reference"=w324) -> ("error out"=w332:errorcluster)  [unwired: 7 in, 1 out]
            n169 = Merge Errors(w334, w332) -> (w331:errorcluster)
            n170 = Unbundle By Name(w322) -> ("File Obj"=w321:refnum<class "File.lvclass">, "View File"=w319:bool)
            n171 = call "Error Reported.vi"("Error"=w331) -> ()  [unwired: 10 in, 1 out]
            n172 = case shown="True" w319 {
              tunnel: w321 -> [w337 w339]
              tunnel: [w337 w338] -> w320
              frame False {
              }
              frame True {
                n173 = call-dynamic "View File.vi"("File in"=w339) -> ("File out"=w338:refnum<class "File.lvclass">)  [unwired: 9 in, 1 out]
              }
            }
            n174 = call-dynamic "Close File.vi"("File in"=w320) -> ()  [unwired: 9 in, 2 out]
          }
          frame Default {
            # "'Default' case only runs if there is a message that isn't defined in any of the other cases.  Output a programming error."
            n175 = call "Module Name--constant.vi"() -> ("Module Name"=w344:string)  [unwired: 11 in]
            n176 = Format Into String(format string="The invalid message string \"%s\" was received in the Message Handling Loop for module \"%s\".", w345, w344) -> (resulting string=w340:string)  [unwired: 2 in, 1 out]
            n177 = call <vilib>:"Error Cluster From Error Code.vi"("show call chain? (False)"=TRUE, "error message (\"\")"=w340, "error code (0)"=1) -> ("error out"=w347:errorcluster)  [unwired: 6 in]
            n178 = Merge Errors(w348, w347) -> (w349:errorcluster)
          }
        }
        n179 = call-dynamic "Delacor_lib_QMH_Error Handler - Message Handling Loop.vi"("error in"=w135, "Message Queue in"=w134) -> ("dup error in"=w136:errorcluster)  [unwired: 8 in, 1 out]
      }
    }
    frame Error {
      # "Synchronize Caller Events.vi will inform Start Module.vi that the module has launched and will let the code calling Start Module.vi register for broadcasts and would permit the caller receive the broadcast that an error occurred at launch time."
      n180 = call-dynamic "Delacor_lib_QMH_Release Message Queue.vi"("error in"=w357, "Message Queue"=w350) -> ("error out"=w356:errorcluster)  [unwired: 9 in]
      n181 = call "Synchronize Caller Events.vi"("Singleton Module Admin in"=w351) -> ("error out"=w358:errorcluster)  [unwired: 9 in, 1 out]
      n182 = call "Module Name--constant.vi"() -> ("Module Name"=w354:string)  [unwired: 11 in]
      n183 = Format Into String(format string="An error occurred during initialization. %s is no longer running.", w354) -> (resulting string=w352:string)  [unwired: 2 in, 1 out]
      n184 = Merge Errors(w356, w358) -> (w359:errorcluster)
      n185 = call "Error Reported.vi"("Additional Information"=w352, "Error"=w359) -> ()  [unwired: 9 in, 1 out]
    }
  }
  n186 = Merge Errors(w14, w17) -> (w13:errorcluster)
  n187 = call "Close Module.vi"("error in"=w13, "Module Admin in"=w8) -> ("error out"=w15:errorcluster, "External Launch"=w1:bool, "Module Admin out"=w2:refnum<class "Delacor_lib_QMH_Module Admin.lvclass">)  [unwired: 7 in]
  n188 = Unregister For Events(event registration refnum=w7, error in=w15) -> (error out=w12:errorcluster)
  "error out" <- w12
  n189 = case "External Launch?" shown="True" w1 {
    tunnel: w12 -> [_ w360]
    frame False {
    }
    frame True {
      n190 = case shown="No Error" w360 {
        frame No Error {
          n191 = invoke on="Invoke Node" class="VI" method="FP.Close"() -> ()  [unwired: 3 in, 3 out]
        }
        frame Error {
          n192 = disable-structure shown="Default" {
            frame condition #0 (active) {
              n193 = invoke class="VI" method="FP.Open"("Activate"=TRUE ("Activate?")) -> ()  [unwired: 4 in, 5 out]
            }
            frame condition #1 {
              # "Don't show panel on error if running inside a built EXE."
            }
          }
        }
      }
    }
  }
  n194 = local write "Module Admin"(w2) -> ()
